vi "GC EX CMS Vacuum - Step 3.vi"(7 "Step":i32, 8 "error in":errorcluster, 9 "Test Results In":T8, 10 "Gas":T1, 11 "GC Configuration":T2) -> (0 "error out":errorcluster, 1 "Test Results Out":T8, 2 "Gas Out":T1 caption="Gas", 3 "GC Configuration Out":T2)   [LabVIEW 2015]
uses:
  Controls/Test Information.ctl
  Controls/Vacuum Test.ctl
  Controls/Test Timing.ctl
  Controls/Vaccum Thresholds.ctl
  Controls/Helium Test.ctl
  Controls/Helium Thresholds.ctl
  CAN Communication/Gas/Typedefs/Session Handle.ctl
  CAN Communication/Gas/Gas.lvclass
  Controls/Test Results.ctl
  Controls/Step Result.ctl
  CAN Communication/Gas/Typedefs/Valves.ctl
  SubVIs/Timing/Timing.lvlib
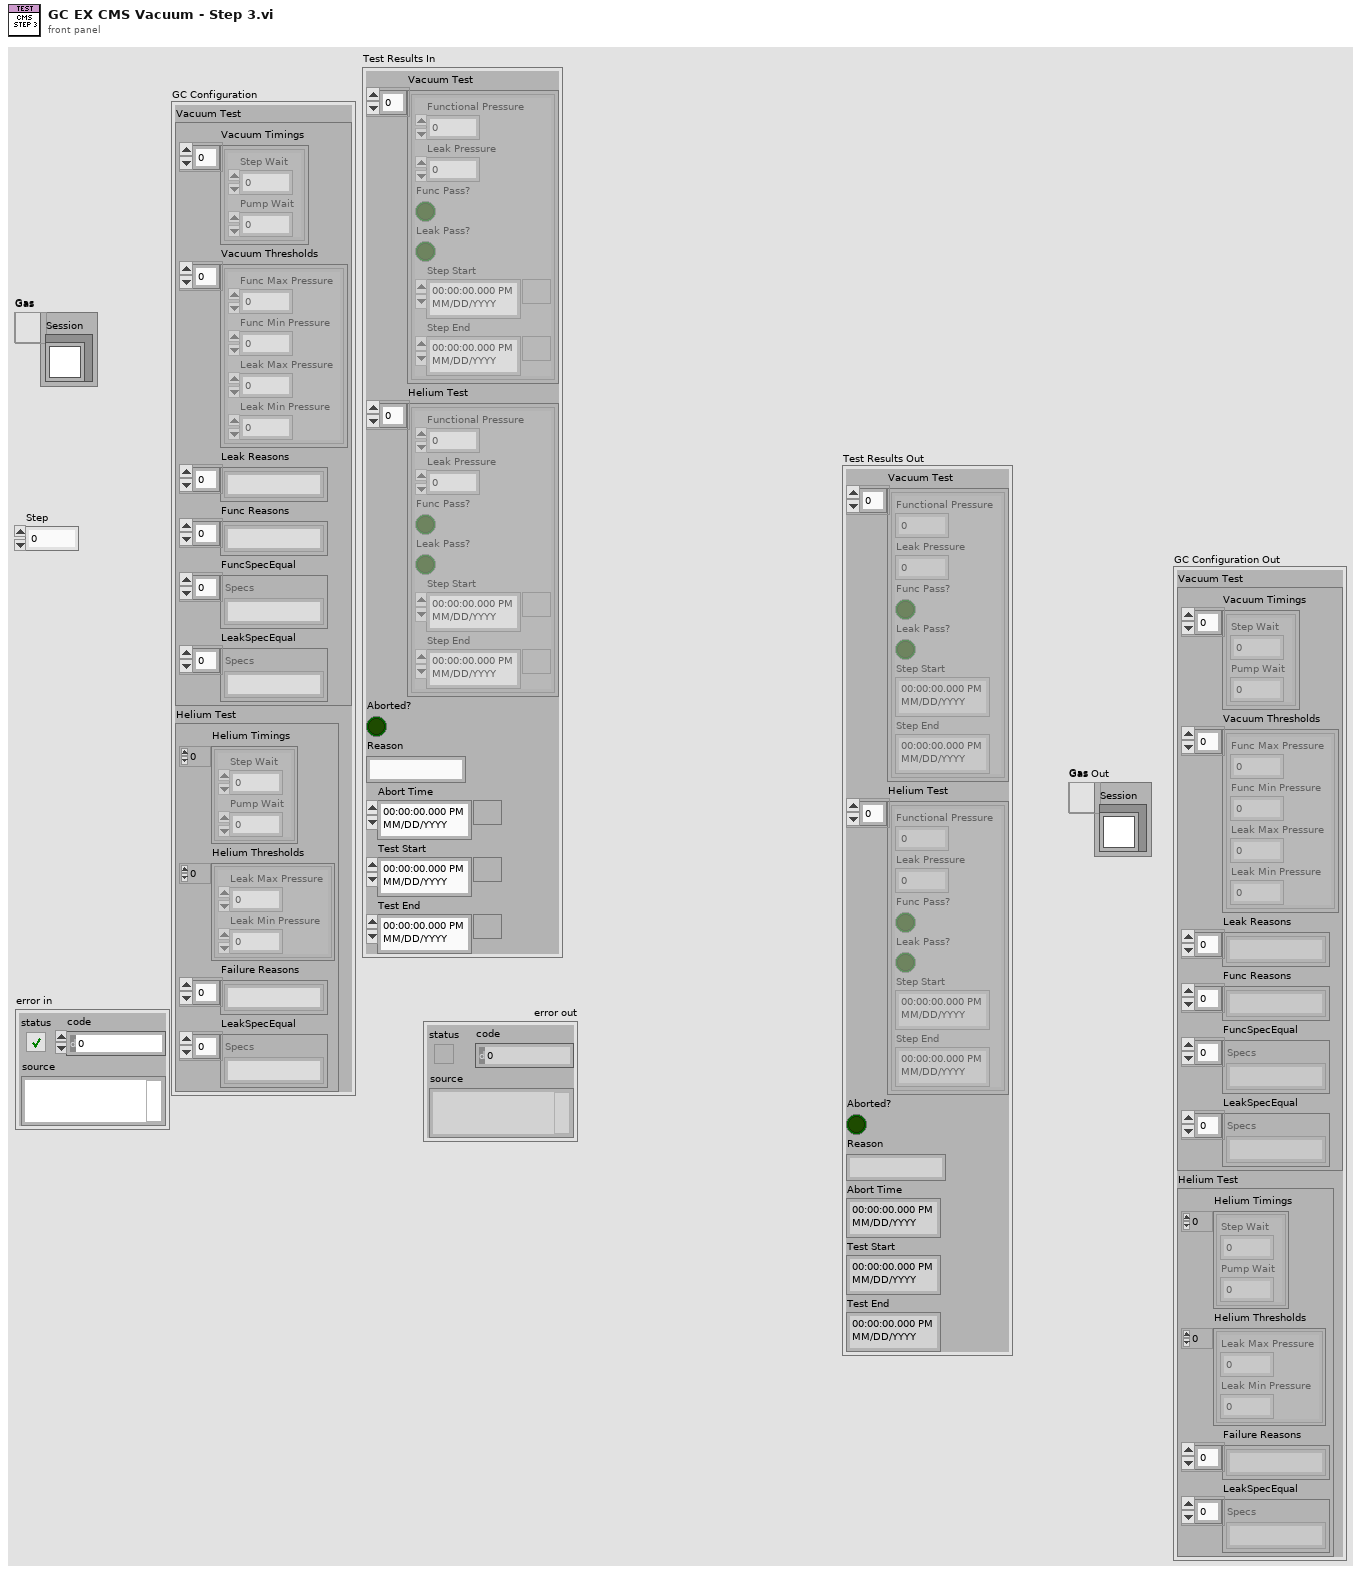
[diagram p1: front panel]
types:
  T1 = typedef "Gas.lvclass/Session Handle.ctl" = refnum<data-value>
  T2 = typedef "Test Information.ctl" = cluster{"Vacuum Test":T3, "Helium Test":T6}
  T3 = typedef "Vacuum Test.ctl" = cluster{"Vacuum Timings":T4[], "Vacuum Thresholds":T5[], "Leak Reasons":string[], "Func Reasons":string[], "FuncSpecEqual":string[], "LeakSpecEqual":string[]}
  T4 = typedef "Test Timing.ctl" = cluster{"Step Wait":dbl, "Pump Wait":dbl}
  T5 = typedef "Vaccum Thresholds.ctl" = cluster{"Func Max Pressure":dbl, "Func Min Pressure":dbl, "Leak Max Pressure":dbl, "Leak Min Pressure":dbl}
  T6 = typedef "Helium Test.ctl" = cluster{"Helium Timings":T4[], "Helium Thresholds":T7[], "Failure Reasons":string[], "LeakSpecEqual":string[]}
  T7 = typedef "Helium Thresholds.ctl" = cluster{"Leak Max Pressure":dbl, "Leak Min Pressure":dbl}
  T8 = typedef "Test Results.ctl" = cluster{"Vacuum Test":T9[], "Helium Test":T9[], "Aborted?":bool, "Reason":string, "Abort Time":timestamp, "Test Start":timestamp, "Test End":timestamp}
  T9 = typedef "Step Result.ctl" = cluster{"Functional Pressure":dbl, "Leak Pressure":dbl, "Func Pass?":bool, "Leak Pass?":bool, "Step Start":timestamp, "Step End":timestamp}
  T10 = typedef "Gas.lvclass/Valves.ctl" = u16
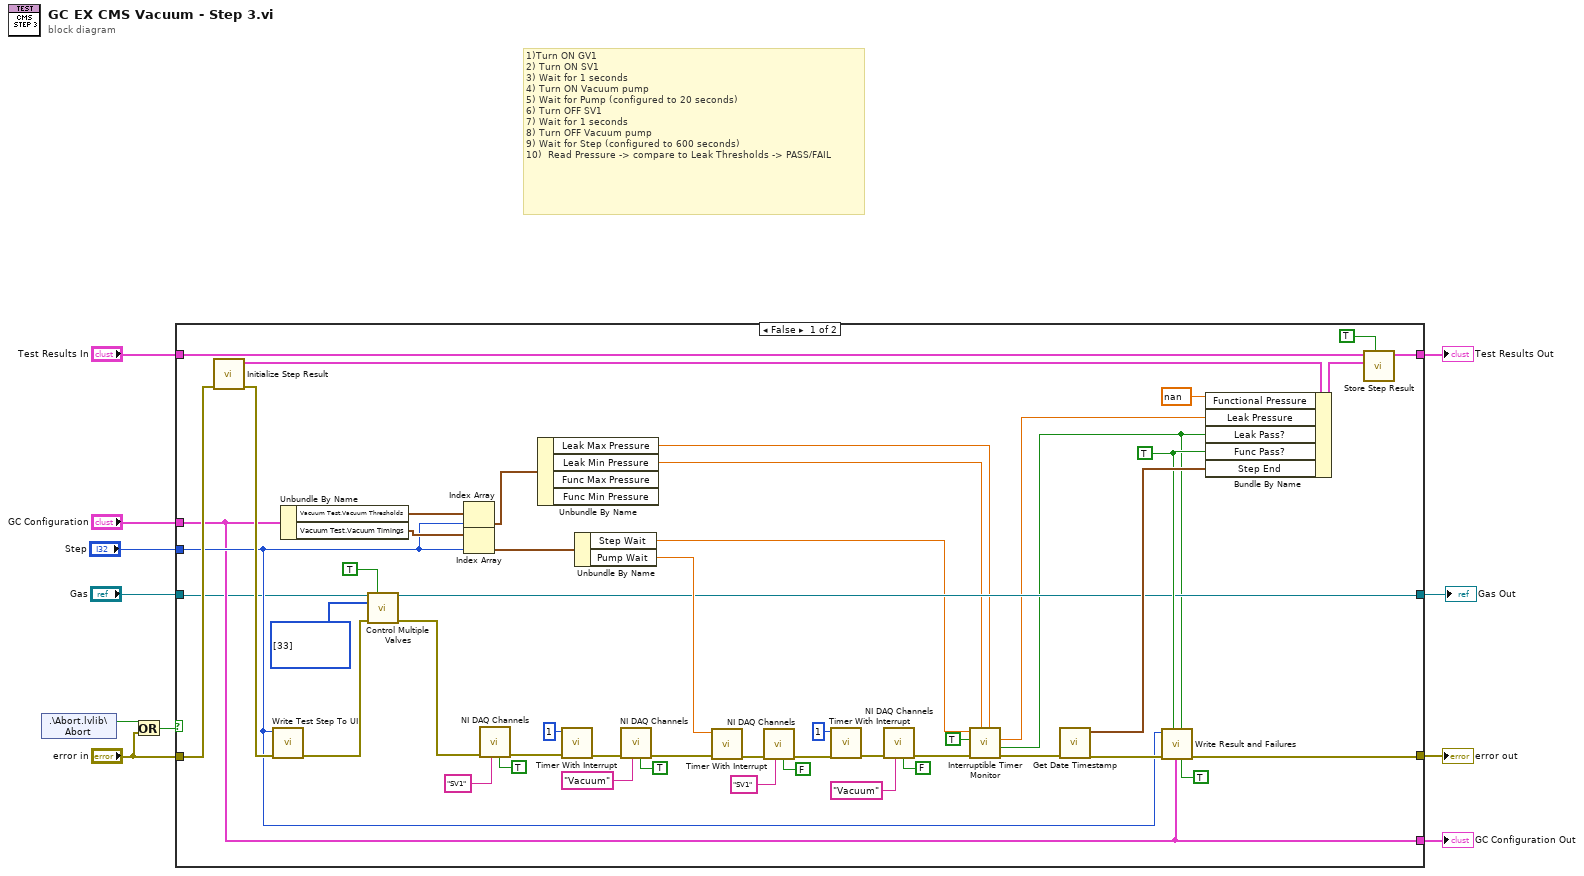
[diagram p0: block diagram]
diagram:
  # "1)Turn ON GV1\n2) Turn ON SV1\n3) Wait for 1 seconds\n4) Turn ON Vacuum pump\n5) Wait for Pump (configured to 20 seconds)\n6) Turn OFF SV1\n7) Wait for 1 seconds\n8) Turn OFF Vacuum pump\n9) Wait for Step (configured to 600 seconds)\n10)  Read Pressure -> compare to Leak Thresholds -> PASS/FAIL"
  n1 = shared-variable ".\\Abort.lvlib\\Abort"() -> (w10:bool)  [unwired: 1 in, 1 out]
  n2 = Or(x=w10, y="error in") -> (x .or. y?=w9:bool)
  n3 = case shown="False" w9 {
    tunnel: "error in" -> [w61 w64]
    tunnel: "Test Results In" -> [w58 w65]
    tunnel: [w59 w65] -> w7
    tunnel: [w49 w64] -> w6
    tunnel: "GC Configuration" -> [w47 w63]
    tunnel: "Step" -> [w48 _]
    tunnel: [w47 w63] -> w3
    tunnel: [w37 w62] -> w1
    tunnel: "Gas" -> [w43 w62]
    frame False {
      w38 = TRUE ("Func Pass?")
      w42 = T10[] [33] items=["GV1"=33, "GV2"=34, "GV3"=35, "GV4"=36, "GV5"=37, "GV6"=38, "GV7"=39, "GV8"=40, "GV9"=41, "GV10"=42, "GV11"=43, "LV3"=51, "LV4"=52] ("Valves")
      n4 = call "Initialize Step Result.vi"("error in (no error)"=w61) -> ("error out"=w60:errorcluster, "New Step Result"=w57:T9)  [unwired: 8 in, 1 out]
      n5 = call "Write Test Step To UI.vi"("error in (no error)"=w60, "Step"=w48) -> ("error out"=w40:errorcluster)  [unwired: 9 in]
      n6 = Unbundle By Name(w47) -> ("Vacuum Test.Vacuum Thresholds"=w54:T5[], "Vacuum Test.Vacuum Timings"=w53:T4[])
      n7 = call "Control Multiple Valves.vi"("Session Handle in"=w43, "Energize?"=TRUE, "Valves"=w42, "error in (no error)"=w40) -> ("Session Handle out"=w37:T1, "error out"=w34:errorcluster)  [unwired: 8 in, 2 out]
      n8 = Index Array(array=w54, index=w48) -> (element=w51:T5)
      n9 = Index Array(array=w53, index=w48) -> (element=w52:T4)
      n10 = call "NI DAQ Channels.vi"("Control"=TRUE ("State"), "Channel"="SV1", "error in (no error)"=w34) -> ("error out"=w33:errorcluster)  [unwired: 7 in, 1 out]
      n11 = Unbundle By Name(w51) -> ("Leak Max Pressure"=w19:dbl, "Leak Min Pressure"=w20:dbl)  [unwired: 2 out]
      n12 = call "Timer With Interrupt.vi"("error in (no error)"=w33, "Wait (s)"=1) -> ("error out"=w31:errorcluster)  [unwired: 7 in, 2 out]
      n13 = Unbundle By Name(w52) -> ("Step Wait"=w22:dbl, "Pump Wait"=w45:dbl)
      n14 = call "NI DAQ Channels.vi"("Control"=TRUE ("State"), "Channel"="Vacuum", "error in (no error)"=w31) -> ("error out"=w30:errorcluster)  [unwired: 7 in, 1 out]
      n15 = call "Timer With Interrupt.vi"("error in (no error)"=w30, "Wait (s)"=w45) -> ("error out"=w28:errorcluster)  [unwired: 7 in, 2 out]
      n16 = call "NI DAQ Channels.vi"("Control"=FALSE ("State"), "Channel"="SV1", "error in (no error)"=w28) -> ("error out"=w27:errorcluster)  [unwired: 7 in, 1 out]
      n17 = call "Timer With Interrupt.vi"("error in (no error)"=w27, "Wait (s)"=1) -> ("error out"=w25:errorcluster)  [unwired: 7 in, 2 out]
      n18 = call "NI DAQ Channels.vi"("Control"=FALSE ("State"), "Channel"="Vacuum", "error in (no error)"=w25) -> ("error out"=w23:errorcluster)  [unwired: 7 in, 1 out]
      n19 = call "Interruptible Timer Monitor.vi"("Max"=w19, "Min"=w20, "error in (no error)"=w23, "Update UI?"=TRUE, "Wait (s)"=w22) -> ("error out"=w17:errorcluster, "In Range?"=w16:bool, "Leak Rate"=w18:dbl)  [unwired: 2 in, 2 out]
      n20 = call "Get Date Timestamp.vi"("error in (no error)"=w17) -> ("error out"=w50:errorcluster, "current time"=w55:timestamp)  [unwired: 9 in]
      n21 = call "Write Result and Failures.vi"("Vacuum?"=TRUE, "Leak"=w16, "GC Configuration"=w47, "Func"=w38, "error in (no error)"=w50, "Step"=w48) -> ("error out"=w49:errorcluster)  [unwired: 5 in]
      n22 = Bundle By Name(cluster=w57, "Functional Pressure"=nan, "Leak Pressure"=w18, "Leak Pass?"=w16, "Func Pass?"=w38, "Step End"=w55) -> (w56:T9)
      n23 = call "Store Step Result.vi"("Vacuum?"=TRUE, "Step Result"=w56, "Test Results In"=w58) -> ("Test Results Out"=w59:T8)  [unwired: 8 in]
    }
    frame True {
    }
  }
  "error out" <- w6
  "Test Results Out" <- w7
  "GC Configuration Out" <- w3
  "Gas Out" <- w1
